vi "Is Created Queue.vi"(10 "Created Queue Alias":string, 11 "Base Queue jettl in":refnum<class "Base Queue jettl.lvclass">) -> (2 "Is Created Queue?":bool, 3 "Base Queue jettl out":refnum<class "Base Queue jettl.lvclass">)   [LabVIEW 2021, in "jettl.lvlib" / "Base Queue jettl.lvlib" / "Base Queue jettl.lvclass"]
uses:
  Base Queue jettl.lvclass
  Base Queue jettl.lvclass/Base Queue jettl.ctl
  Queue Mailbox/Queue Mailbox.lvlib
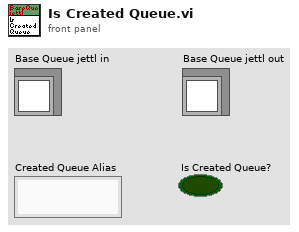
[diagram p1: front panel]
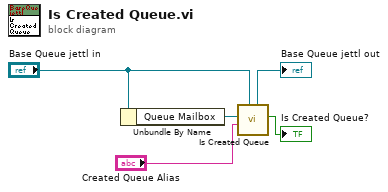
[diagram p0: block diagram]
diagram:
  n1 = Unbundle By Name("Base Queue jettl in") -> ("Queue Mailbox"=w5:refnum<data-value>)
  n2 = call "Is Created Queue.vi"("jettl in"="Base Queue jettl in", "Created Queue Alias"="Created Queue Alias", "Queue Mailbox"=w5) -> ("Is Created Queue?"=→"Is Created Queue?":bool, "jettl out"=→"Base Queue jettl out":refnum<class "Base Queue jettl.lvclass">)  [unwired: 7 in]
